vi "Stop Module.vi"(8 "error in":errorcluster, 9 "Wait for Module to stop? (F)":bool, 10 "Origin":string, 11 "Module ID":i32=-1) -> (0 "error out":errorcluster)   [LabVIEW 2025, in "Stepper.lvlib"]
doc: "Send the Stop request to the Module's Main.vi. If <b>Wait for Module to stop?</b> is TRUE, then this VI will not complete execution until the Module Main VI has stopped running.\n\n<b>Note:</b> If the cloneable module is running as singleton, then the 'Wait for Module to stop?' input is ignored... this VI will <b>always</b> wait until a cloneable Main VI running as singleton has stopped running.\n_____\nBased on DQMH Dev Tools: Project Template 7.1.2.1547."
uses:
  Stepper.lvlib
  Stop Argument--cluster.ctl
  Module Running State--enum.ctl
  Main.vi
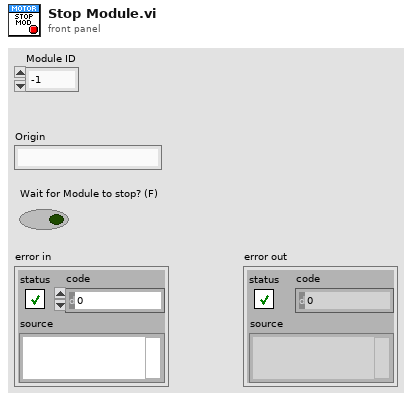
[diagram p1: front panel]
types:
  T1 = typedef "Stepper.lvlib/Module Running State--enum.ctl" = enum16{"Not Running", "Running as Cloneable", "Running as Singleton"}
  T2 = typedef "Stepper.lvlib/Stop Argument--cluster.ctl" = cluster{"Module ID":i32, "Origin":string, "Exit via Stop Module Req?":bool, "Wait for Module to stop?":bool}
  T3 = typedef "Stepper.lvlib/Request Events--cluster.ctl" = cluster{"Stop Module":refnum<user-event>, "Show Panel":refnum<user-event>, "Hide Panel":refnum<user-event>, "Show Diagram":refnum<user-event>, "Get Module Execution Status":refnum<user-event>}
  T4 = enum32{"Bad", "Idle", "Run top level", "Running"}
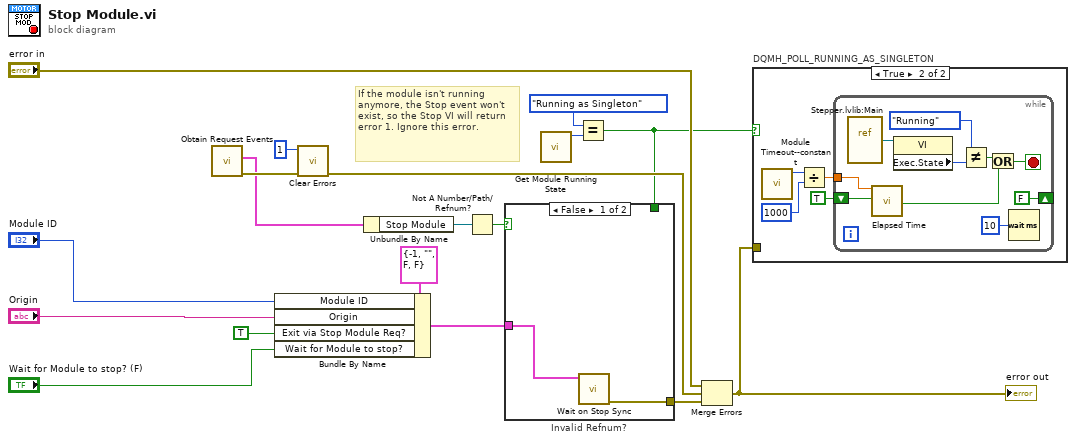
[diagram p0: block diagram]
diagram:
  # "If the module isn't running anymore, the Stop event won't exist, so the Stop VI will return error 1. Ignore this error."
  n1 = call "Obtain Request Events.vi"() -> ("error out"=w12:errorcluster, "Stepper Request Events"=w10:T3)  [unwired: 10 in]
  n2 = Bundle By Name(cluster=T2 {"Module ID"=-1, "Origin"="", "Exit via Stop Module Req?"=FALSE, "Wait for Module to stop?"=FALSE} ("event data"), "Module ID"="Module ID", "Origin"="Origin", "Exit via Stop Module Req?"=TRUE, "Wait for Module to stop?"="Wait for Module to stop? (F)") -> (w13:T2)
  n3 = call <vilib>:"Clear Errors.vi"("error in (no error)"=w12, "specific error code to clear (0: all)"=1) -> ("error out"=w9:errorcluster)  [unwired: 4 in, 1 out]
  n4 = Unbundle By Name(w10) -> ("Stop Module"=w14:refnum<user-event>)
  n5 = Not A Number/Path/Refnum?(number/path/refnum=w14) -> (NaN/Path/Refnum?=w15:bool)
  n6 = call "Get Module Running State.vi"() -> ("Module Running State"=w5:T1)  [unwired: 11 in]
  n7 = Equal?(x=Module_Running_State--enum."Running as Singleton", y=w5) -> (x = y?=w4:bool)
  n8 = case "Invalid Refnum?" shown="False" w15 {
    tunnel: [w20 _] -> w8
    tunnel: w13 -> [w19 _]
    tunnel: w4 -> [_ _]
    frame False {
      n9 = call "Wait on Stop Sync.vi"("Stop Argument"=w19) -> ("error out"=w20:errorcluster)  [unwired: 10 in]
    }
    frame True {
      # "Module is exiting. No need to send the standard \"not running\" error that is sent in other request VIs."
    }
  }
  n10 = Merge Errors("error in", w9, w8) -> (w2:errorcluster)
  "error out" <- w2
  n11 = case "DQMH_POLL_RUNNING_AS_SINGLETON" shown="True" w4 {
    tunnel: w2 -> [_ _]
    frame False {
    }
    frame True {
      n12 = call "Module Timeout--constant.vi"() -> ("Module Timeout"=w24:i32)  [unwired: 11 in]
      n13 = Divide(x=w24, y=1000) -> (x/y=w22:dbl)
      n14 = while {
        tunnel: w22 -> [w27]
        shift-right: [FALSE] -> _
        shift-left: TRUE -> [w28]
        stop <- w30 stop-if-true
        n15 = vi-ref "Stepper.lvlib:Main.vi"() -> (w34:refnum<vi>)
        n16 = call "Elapsed Time"("Time Target (s)"=w27, "Reset"=w28) -> ("Time has Elapsed"=w26:bool)  [unwired: 10 in, 7 out]
        n17 = property class="VI"(reference=w34) -> ("Exec.State"=w33:T4)  [unwired: 1 in, 2 out]
        n18 = Not Equal?(x=T4."Running", y=w33) -> (x != y?=w31:bool)
        n19 = Or(x=w31, y=w26) -> (x .or. y?=w30:bool)
        n20 = Wait (ms)(milliseconds to wait=u32 10) -> ()  [unwired: 1 out]
      }
    }
  }
